vi "GetType.vi"(8 "error in (no error)":errorcluster, 11 "Move Msg":refnum<class "Move Msg.lvclass">) -> (0 "error out":errorcluster, 2 "Data Sample":variant, 3 "Move Msg":refnum<class "Move Msg.lvclass">)   [LabVIEW 2016, in "CS++Motor.lvlib" / "Move Msg.lvclass"]
uses:
  Move Msg.lvclass
  Move Msg.lvclass/Move Msg.ctl
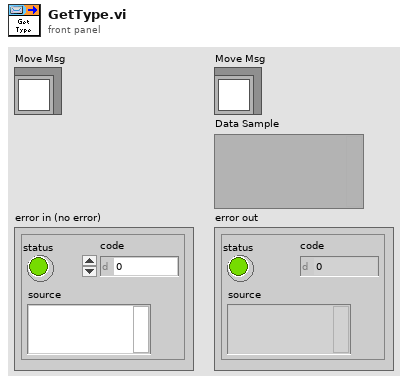
[diagram p1: front panel]
types:
  T1 = cluster{"AxisNumber":u8, "Position":dbl, "Relative?":bool}
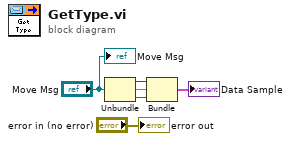
[diagram p0: block diagram]
diagram:
  n1 = Unbundle("Move Msg") -> (w3:u8, w2:dbl, w1:bool)
  n2 = Bundle("AxisNumber"=w3, "Position"=w2, "Relative?"=w1) -> (→"Data Sample":T1)  [unwired: 1 in]
  "error out" <- "error in (no error)"
  "Move Msg" <- "Move Msg"
